vi "System4.vi"() -> ()   [LabVIEW 2013]
uses:
  <vilib>/imath/engines/lvmath/Plug In/_Char/NIMS_CH_character datatype.ctl
  <vilib>/imath/engines/lvmath/Functions/Error Handling/error.ctl
  <vilib>/Analysis/2dsp.llb/Complex FFT.vi
  <vilib>/Analysis/3filter.llb/Equi-Ripple HighPass (DBL).vi
  <instrlib>/niUSRP/niUSRP Fetch Rx Data (CDB).vi
  <vilib>/imath/engines/lvmath2/RunTimeEngine/ErrorHandling/NIMS_Finalize Error.vi
  <vilib>/imath/engines/lvmath2/RunTimeEngine/Managers/WorkSpace/UID Generator.vi
  <vilib>/imath/engines/lvmath2/RunTimeEngine/BuiltInFunctions/length/NIMS_length(GV).vi
  <instcachedir>/0/NIMS_length(GV)_08A3D13377FD4E4B96F5795FBF3698FA.lvgen/NIMS_length(GV)_08A3D13377FD4E4B96F5795FBF3698FA_001.vi
  <vilib>/imath/engines/lvmath2/RunTimeEngine/RangeToken/NIMS_Range_R2 - Integer.vi
  <instcachedir>/0/NIMS_Range_R2 - Integer_C51C130E5EA5464EA148B28CDAB9615A.lvgen/NIMS_Range_R2 - Integer_C51C130E5EA5464EA148B28CDAB9615A_000.vi
  <vilib>/imath/engines/lvmath2/RunTimeEngine/Managers/SymbolTable/Clear UID.vi
  <vilib>/imath/engines/lvmath2/RunTimeEngine/NodeEndStatement/NIMS_NodeEndStatement_Output.vi
  <instcachedir>/0/NIMS_NodeEndStatement_Output_53EC0D466D134D7ABD903AC30B43404B.lvgen/NIMS_NodeEndStatement_Output_53EC0D466D134D7ABD903AC30B43404B_014.vi
  <instcachedir>/0/NIMS_NodeEndStatement_Output_53EC0D466D134D7ABD903AC30B43404B.lvgen/NIMS_NodeEndStatement_Output_53EC0D466D134D7ABD903AC30B43404B_011.vi
  <vilib>/imath/engines/lvmath2/RunTimeEngine/IndexRead/NIMS V(S).vi
  <instcachedir>/0/NIMS V(S)_0488751826AF41519A22953C041130DC.lvgen/NIMS V(S)_0488751826AF41519A22953C041130DC_005.vi
  <vilib>/imathl/engines/lvmath/Functions/Error Handling/Create Error.vi
  <vilib>/imath/engines/lvmath2/RunTimeEngine/BuiltInFunctions/figure/NIMS_figure(I32).vi
  <vilib>/imath/engines/lvmath/Plug In/_Char/NIMS_CH_Character RV to String.vi
  <vilib>/imath/engines/lvmath2/RunTimeEngine/BuiltInFunctions/plot/NIMS_plot(G, Str).vi
  <instcachedir>/0/NIMS_plot(G, Str)_30D49D8623E0484DBD39D394DDFCBE95.lvgen/NIMS_plot(G, Str)_30D49D8623E0484DBD39D394DDFCBE95_000.vi
  <vilib>/imath/engines/lvmath2/RunTimeEngine/NonStaticBuiltInFunctions/Manual/NIMS_NS_load.vi
  <vilib>/imath/engines/lvmath2/RunTimeEngine/RunTimeType/NIMS_RunTimeType_From StrictType (excl LVString).vi
  <instcachedir>/0/NIMS_RunTimeType_From StrictType (excl LVString)_4DEE718D6EB74582AA20236969C084FC.lvgen/NIMS_RunTimeType_From StrictType (excl LVString)_4DEE718D6EB74582AA20236969C084FC_000.vi
  <vilib>/imath/engines/lvmath2/RunTimeEngine/Managers/SymbolTable/Write Variable.vi
  <vilib>/imath/engines/lvmath2/RunTimeEngine/RowToken/NIMS_RowToken-nonstatic.vi
  <vilib>/imath/engines/lvmath2/RunTimeEngine/MatrixToken/NIMS_MatrixToken-nonstatic.vi
  <vilib>/imath/engines/lvmath2/RunTimeEngine/RunTimeSymbolToken/NIMS_RunTimeSymbolToken_ReadVariable-1out.vi
  <vilib>/imath/engines/lvmath/Functions/Error Handling/MergeErrorsWrapper.vi
  <vilib>/imath/engines/lvmath2/RunTimeEngine/LocalVariableDefStatement/MC_LocalVariableDefStatement_Display.vi
  <vilib>/imath/engines/lvmath2/RunTimeEngine/RunTimeSymbolToken/NIMS_RunTimeSymbolToken_ResolveSymbol.vi
  <instcachedir>/0/NIMS_RunTimeSymbolToken_ResolveSymbol_F94DACEDB8D84373A3303A9E667D843C.lvgen/NIMS_RunTimeSymbolToken_ResolveSymbol_F94DACEDB8D84373A3303A9E667D843C_003.vi
  <vilib>/imath/engines/lvmath2/RunTimeEngine/CommandStatement/NIMS_CommandStatement_MaskErr.vi
  <vilib>/imath/engines/lvmath2/RunTimeEngine/Managers/SymbolTable/Read Variable.vi
  <vilib>/imath/engines/lvmath2/RunTimeEngine/RunTimeType/NIMS_RunTimeType_Get Case Value.vi
  <vilib>/imath/engines/lvmath2/RunTimeEngine/NodeEndStatement/MC_NodeEndStatement_Dispose.vi
  <instcachedir>/0/NIMS_NodeEndStatement_Output_53EC0D466D134D7ABD903AC30B43404B.lvgen/NIMS_NodeEndStatement_Output_53EC0D466D134D7ABD903AC30B43404B_004.vi
  <vilib>/imath/engines/lvmath2/RunTimeEngine/RunTimeType/NIMS_RunTimeType_To Numeric.vi
  <instcachedir>/0/NIMS_RunTimeType_To Numeric_4795FB10E831402FABFA341B47E20681.lvgen/NIMS_RunTimeType_To Numeric_4795FB10E831402FABFA341B47E20681_000.vi
  <vilib>/imath/engines/lvmath2/RunTimeEngine/NodeEndStatement/NIMS_NodeEndStatement_Get Vector.vi
  <instcachedir>/0/NIMS_NodeEndStatement_Get Vector_BE4364D373AE46158CA0B14DEB6F98C8.lvgen/NIMS_NodeEndStatement_Get Vector_BE4364D373AE46158CA0B14DEB6F98C8_003.vi
  <vilib>/imath/engines/lvmath/Plug In/_Char/RunTimeType/NIMS_CH_RunTimeType_To Character 2D.vi
  <instcachedir>/0/NIMS_NodeEndStatement_Get Vector_BE4364D373AE46158CA0B14DEB6F98C8.lvgen/NIMS_NodeEndStatement_Get Vector_BE4364D373AE46158CA0B14DEB6F98C8_000.vi
  <vilib>/imath/engines/lvmath/Plug In/_Char/NIMS_CH_Character 1D to U8 1D.vi
  <instcachedir>/0/NIMS_NodeEndStatement_Output_53EC0D466D134D7ABD903AC30B43404B.lvgen/NIMS_NodeEndStatement_Output_53EC0D466D134D7ABD903AC30B43404B_000.vi
  <instcachedir>/0/NIMS_NodeEndStatement_Output_53EC0D466D134D7ABD903AC30B43404B.lvgen/NIMS_NodeEndStatement_Output_53EC0D466D134D7ABD903AC30B43404B_001.vi
  <instcachedir>/0/NIMS_length(GV)_08A3D13377FD4E4B96F5795FBF3698FA.lvgen/NIMS_length(GV)_08A3D13377FD4E4B96F5795FBF3698FA_002.vi
  <vilib>/imath/engines/lvmath2/RunTimeEngine/IndexRead/NIMS V(R2).vi
  <instcachedir>/0/NIMS V(R2)_C76619605A0E4E9F8B2FA9389712AC47.lvgen/NIMS V(R2)_C76619605A0E4E9F8B2FA9389712AC47_001.vi
  <vilib>/imath/engines/lvmath2/RunTimeEngine/BuiltInFunctions/angle/NIMS_angle.vi
  <instcachedir>/0/NIMS_angle_6DDAE2BD99E0421EB990B6436E94D88F.lvgen/NIMS_angle_6DDAE2BD99E0421EB990B6436E94D88F_005.vi
  <vilib>/imath/engines/lvmath2/RunTimeEngine/RangeToken/NIMS_Range.vi
  <instcachedir>/0/NIMS_Range_7481B155BEE341ECA0F59DDB444E2C09.lvgen/NIMS_Range_7481B155BEE341ECA0F59DDB444E2C09_001.vi
  <vilib>/imath/engines/lvmath2/RunTimeEngine/IndexRead/NIMS V(V).vi
  <instcachedir>/0/NIMS V(V)_298D9CB7BFEB42B8BC8D9C3C28AE8C70.lvgen/NIMS V(V)_298D9CB7BFEB42B8BC8D9C3C28AE8C70_000.vi
  <vilib>/imath/engines/lvmath2/RunTimeEngine/BuiltInFunctions/mean/NIMS_CS=mean(CV,I32).vi
  <instcachedir>/0/NIMS_angle_6DDAE2BD99E0421EB990B6436E94D88F.lvgen/NIMS_angle_6DDAE2BD99E0421EB990B6436E94D88F_003.vi
  <vilib>/imath/engines/lvmath2/RunTimeEngine/ErrorHandling/NIMS_Create Error From Enums.vi
  <vilib>/imath/engines/lvmath2/RunTimeEngine/BuiltInFunctions/mean/NIMS_RS=mean(RV,I32).vi
  <vilib>/imath/engines/lvmath2/RunTimeEngine/BuiltInFunctions/abs/NIMS_abs(signed).vi
  <instcachedir>/0/NIMS_abs(signed)_C4FCB8E6058B49B797C7C8D53CA5F6EC.lvgen/NIMS_abs(signed)_C4FCB8E6058B49B797C7C8D53CA5F6EC_000.vi
  <vilib>/imath/engines/lvmath2/RunTimeEngine/BuiltInFunctions/linramp/NIMS_linramp.vi
  <vilib>/imath/engines/lvmath2/RunTimeEngine/ArithmeticOperatorToken/NIMS_ArithmeticOperator_plus.vi
  <instcachedir>/0/NIMS_ArithmeticOperator_plus_8A46DAFC24D445C9B2C97B626139369E.lvgen/NIMS_ArithmeticOperator_plus_8A46DAFC24D445C9B2C97B626139369E_005.vi
  <vilib>/imath/engines/lvmath2/RunTimeEngine/BuiltInFunctions/numelements/NIMS_numelements.vi
  <instcachedir>/0/NIMS_numelements_A776DA77F73142F68C2F209B523114C5.lvgen/NIMS_numelements_A776DA77F73142F68C2F209B523114C5_003.vi
  <vilib>/imath/engines/lvmath2/RunTimeEngine/BuiltInFunctions/zeros/NIMS_V=zeros(I32,I32).vi
  <vilib>/imath/engines/lvmath2/RunTimeEngine/CommandStatement/MC_CommandStatement_break.vi
  LabVIEW Data/MathScriptVIs/MCStatic_31879994332_13cee6d0e2951097849577d15734aa47.vi
  <instcachedir>/0/MCStatic_31879994332_13cee6d0e2951097849577d15734aa47_8B05E9F3DA25454388965366AFABC993.lvgen/MCStatic_31879994332_13cee6d0e2951097849577d15734aa47_8B05E9F3DA25454388965366AFABC993_000.vi
  <vilib>/imath/engines/lvmath2/RunTimeEngine/IndexReplace/NIMS V(S)=S.vi
  <instcachedir>/0/NIMS V(S)=S_66A18068148B4981A312229A93EA5C06.lvgen/NIMS V(S)=S_66A18068148B4981A312229A93EA5C06_001.vi
  <instcachedir>/0/NIMS V(S)=S_66A18068148B4981A312229A93EA5C06.lvgen/NIMS V(S)=S_66A18068148B4981A312229A93EA5C06_000.vi
  <instcachedir>/0/NIMS_plot(G, Str)_30D49D8623E0484DBD39D394DDFCBE95.lvgen/NIMS_plot(G, Str)_30D49D8623E0484DBD39D394DDFCBE95_001.vi
  <vilib>/imath/engines/lvmath2/RunTimeEngine/BuiltInFunctions/title/NIMS_title.vi
  <vilib>/imath/engines/lvmath2/RunTimeEngine/BuiltInFunctions/round/NIMS_round(DBL-S).vi
  <vilib>/imath/engines/lvmath2/RunTimeEngine/BuiltInFunctions/grid/NIMS_grid(Enums).vi
  <instcachedir>/0/NIMS V(S)_0488751826AF41519A22953C041130DC.lvgen/NIMS V(S)_0488751826AF41519A22953C041130DC_000.vi
  <instcachedir>/0/NIMS_abs(signed)_C4FCB8E6058B49B797C7C8D53CA5F6EC.lvgen/NIMS_abs(signed)_C4FCB8E6058B49B797C7C8D53CA5F6EC_001.vi
  <vilib>/imath/engines/lvmath2/RunTimeEngine/BuiltInFunctions/max/1 input/NIMS_max(RV).vi
  <instcachedir>/0/NIMS_max(RV)_237633DB1D604D5BA7001287DF3C7957.lvgen/NIMS_max(RV)_237633DB1D604D5BA7001287DF3C7957_000.vi
  <instcachedir>/0/NIMS_Range_7481B155BEE341ECA0F59DDB444E2C09.lvgen/NIMS_Range_7481B155BEE341ECA0F59DDB444E2C09_000.vi
  <vilib>/imath/engines/lvmath2/RunTimeSupport/NIMS_Error if Not Equal.vi
  <instcachedir>/0/NIMS_Error if Not Equal_902F5D2649E64F5087A1EF57C55C58AB.lvgen/NIMS_Error if Not Equal_902F5D2649E64F5087A1EF57C55C58AB_001.vi
  <vilib>/imath/engines/lvmath2/RunTimeEngine/BuiltInFunctions/repeatmx/NIMS_repeatmx(GM, I32, I32).vi
  <instcachedir>/0/NIMS_repeatmx(GM, I32, I32)_71D32CAC8D434697AB9DA7B55FCB46E4.lvgen/NIMS_repeatmx(GM, I32, I32)_71D32CAC8D434697AB9DA7B55FCB46E4_003.vi
  <vilib>/imath/engines/lvmath2/RunTimeEngine/ArithmeticOperatorToken/NIMS_ArithmeticOperator_minus.vi
  <instcachedir>/0/NIMS_ArithmeticOperator_minus_5462A7974F41415E96B34B7C9D041F4F.lvgen/NIMS_ArithmeticOperator_minus_5462A7974F41415E96B34B7C9D041F4F_008.vi
  <instcachedir>/0/NIMS_abs(signed)_C4FCB8E6058B49B797C7C8D53CA5F6EC.lvgen/NIMS_abs(signed)_C4FCB8E6058B49B797C7C8D53CA5F6EC_003.vi
  <vilib>/imath/engines/lvmath2/RunTimeEngine/BuiltInFunctions/min/1 input/NIMS_min(RM).vi
  <instcachedir>/0/NIMS_min(RM)_0DDFAEBC1781439CA067A573026FA64C.lvgen/NIMS_min(RM)_0DDFAEBC1781439CA067A573026FA64C_000.vi
  <vilib>/imath/engines/lvmath2/RunTimeEngine/IndexRead/NIMS M($,V).vi
  <instcachedir>/0/NIMS M($,V)_706F2CE2C8E141269FD4C8A402E169C5.lvgen/NIMS M($,V)_706F2CE2C8E141269FD4C8A402E169C5_004.vi
  <vilib>/imath/engines/lvmath2/RunTimeEngine/IndexReplace/NIMS M($,V)=M.vi
  <instcachedir>/0/NIMS M($,V)=M_DD8F56E7222B4C7AB43CEE6CDE526A04.lvgen/NIMS M($,V)=M_DD8F56E7222B4C7AB43CEE6CDE526A04_003.vi
  <vilib>/imath/engines/lvmath2/RunTimeEngine/IndexRead/NIMS M($).vi
  <instcachedir>/0/NIMS M($)_82D1177398184AFB96A6AFB63C3C3F57.lvgen/NIMS M($)_82D1177398184AFB96A6AFB63C3C3F57_005.vi
  <vilib>/imath/engines/lvmath2/RunTimeEngine/BuiltInFunctions/hold/NIMS_hold(Enums).vi
  <vilib>/imath/engines/lvmath2/RunTimeEngine/BuiltInFunctions/imag/NIMS_imag(Complex).vi
  <instcachedir>/0/NIMS_imag(Complex)_3180D40D00C843A49C2B33397F857BF3.lvgen/NIMS_imag(Complex)_3180D40D00C843A49C2B33397F857BF3_002.vi
  <instcachedir>/0/MCStatic_31879994332_13cee6d0e2951097849577d15734aa47_8B05E9F3DA25454388965366AFABC993.lvgen/MCStatic_31879994332_13cee6d0e2951097849577d15734aa47_8B05E9F3DA25454388965366AFABC993_002.vi
  <vilib>/imath/engines/lvmath2/RunTimeEngine/BuiltInFunctions/crosscorr/NIMS_crosscorr(GV,GV,Str).vi
  <instcachedir>/0/NIMS_crosscorr(GV,GV,Str)_7F516622EB1B4986A7D0F3F178AC2F2E.lvgen/NIMS_crosscorr(GV,GV,Str)_7F516622EB1B4986A7D0F3F178AC2F2E_000.vi
  <instcachedir>/0/NIMS_abs(signed)_C4FCB8E6058B49B797C7C8D53CA5F6EC.lvgen/NIMS_abs(signed)_C4FCB8E6058B49B797C7C8D53CA5F6EC_006.vi
  LabVIEW Data/MathScriptVIs/MCStatic_31879994332_51ed6d19a1ca34c572878de5410fc211.vi
  <instcachedir>/0/MCStatic_31879994332_51ed6d19a1ca34c572878de5410fc211_95B5E1E0CE2B47CE84A8C3844D693930.lvgen/MCStatic_31879994332_51ed6d19a1ca34c572878de5410fc211_95B5E1E0CE2B47CE84A8C3844D693930_000.vi
  <instcachedir>/0/NIMS V(R2)_C76619605A0E4E9F8B2FA9389712AC47.lvgen/NIMS V(R2)_C76619605A0E4E9F8B2FA9389712AC47_002.vi
  <vilib>/imath/engines/lvmath2/RunTimeEngine/ArithmeticOperatorToken/NIMS_ArithmeticOperator_rightdiv(C,C).vi
  <instcachedir>/0/NIMS_ArithmeticOperator_rightdiv(C,C)_088115A0C99E4A54BFBAA9DF92471D5B.lvgen/NIMS_ArithmeticOperator_rightdiv(C,C)_088115A0C99E4A54BFBAA9DF92471D5B_000.vi
  <instcachedir>/0/NIMS_ArithmeticOperator_minus_5462A7974F41415E96B34B7C9D041F4F.lvgen/NIMS_ArithmeticOperator_minus_5462A7974F41415E96B34B7C9D041F4F_016.vi
  <instcachedir>/0/NIMS_abs(signed)_C4FCB8E6058B49B797C7C8D53CA5F6EC.lvgen/NIMS_abs(signed)_C4FCB8E6058B49B797C7C8D53CA5F6EC_007.vi
  <vilib>/imath/engines/lvmath2/RunTimeEngine/BuiltInFunctions/sum/NIMS_sum(GV).vi
  <instcachedir>/0/NIMS_sum(GV)_67F5EC36BC034E54A6BEC5B0673C00E5.lvgen/NIMS_sum(GV)_67F5EC36BC034E54A6BEC5B0673C00E5_000.vi
  MATLAB_func/frequency_synchronisation_sample.m
  MATLAB_func/quadrature_error_correction.m
  <vilib>/imath/engines/lvmath2/RunTimeEngine/Managers/SymbolTable/NIMS_WorkSpace.lvlib
  <vilib>/Analysis/NI_AALPro.lvlib
  <vilib>/Analysis/NI_AALBase.lvlib
  <instcachedir>/0/MCStatic_31879994332_13cee6d0e2951097849577d15734aa47_8B05E9F3DA25454388965366AFABC993.lvgen/MCStatic_31879994332_13cee6d0e2951097849577d15734aa47_8B05E9F3DA25454388965366AFABC993_003.vi
panel:
  out "coerced carrier frequency":dbl=100000.0 format="%#_6p"
  out "Waveform Graph 6":dbl[](graph)
  out "bit_error_rate":dbl
  out "error":dbl
  out "size(s)":i32
  out "length_signal_out":i32
  in  "file (use dialog) 2":path=path "C:/Users/Lab/Downloads/FPGA.3JPG"
  in  "file (use dialog)":path=path "C:/Users/Lab/Downloads/FPGA.JPG"
  out "time":dbl
  out "a":cdb[](array[numeric])
  in  "message number of samples (50000)":i64=50000
  in  "stop 2":bool
  in  "Wakeup #samples (1000)":i64=1000
  out "RX coerced gain":dbl format="%#_6f"
  out "RX coerced IQ rate":dbl=100000.0 format="%#_6p"
  in  "RX gain":dbl format="%#_6f"
  in  "RX IQ rate":dbl=1000000.0 format="%#_6p"
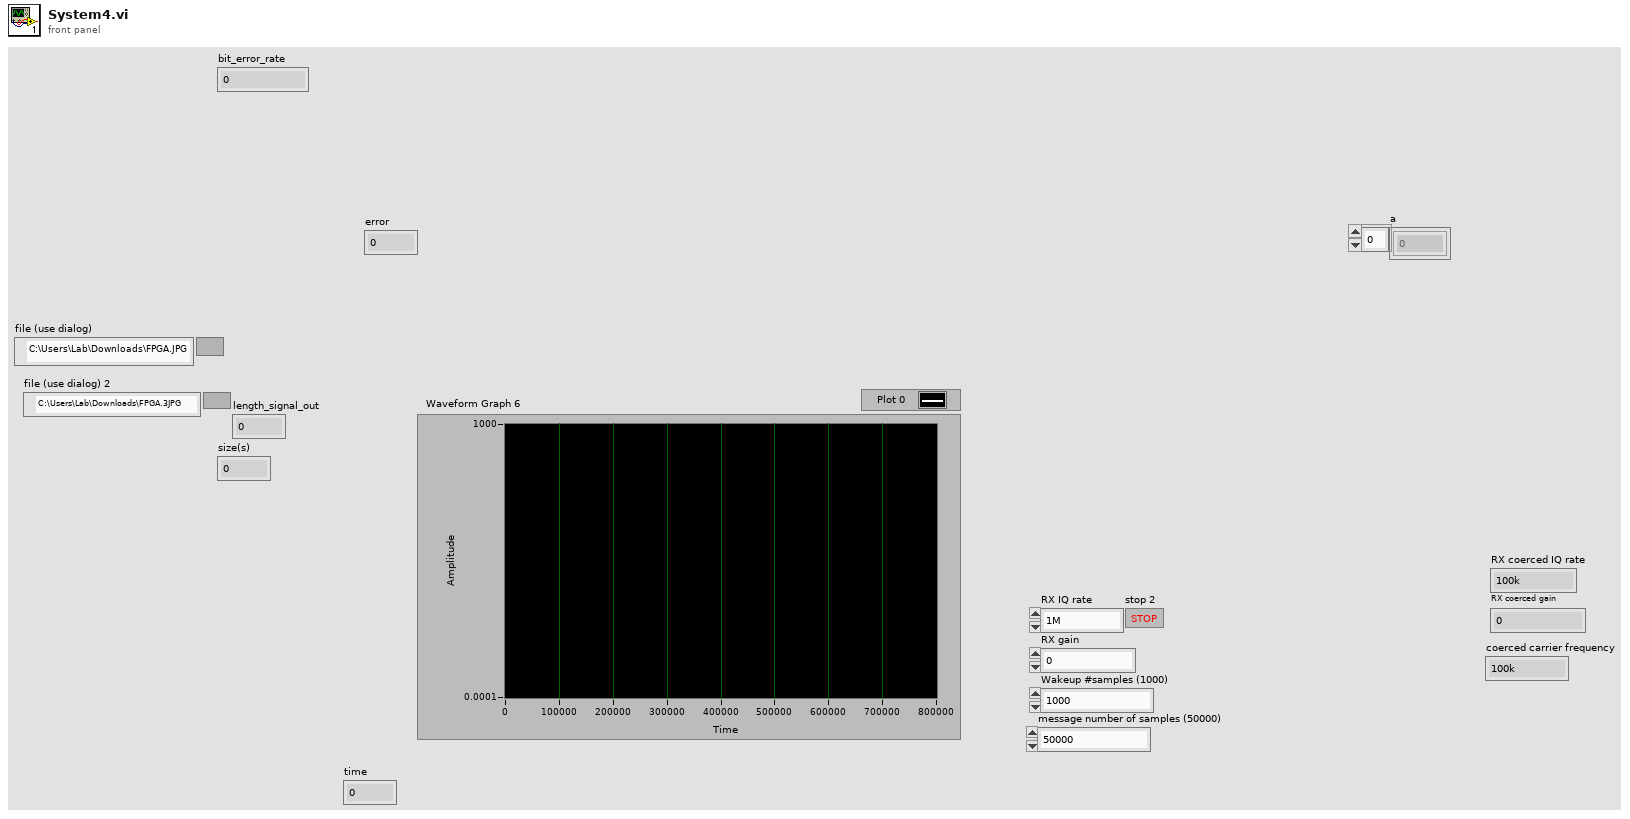
[diagram p1: front panel]
types:
  T1 = typedef "NIMS_CH_character datatype.ctl" = cluster{"Numeric":u8}
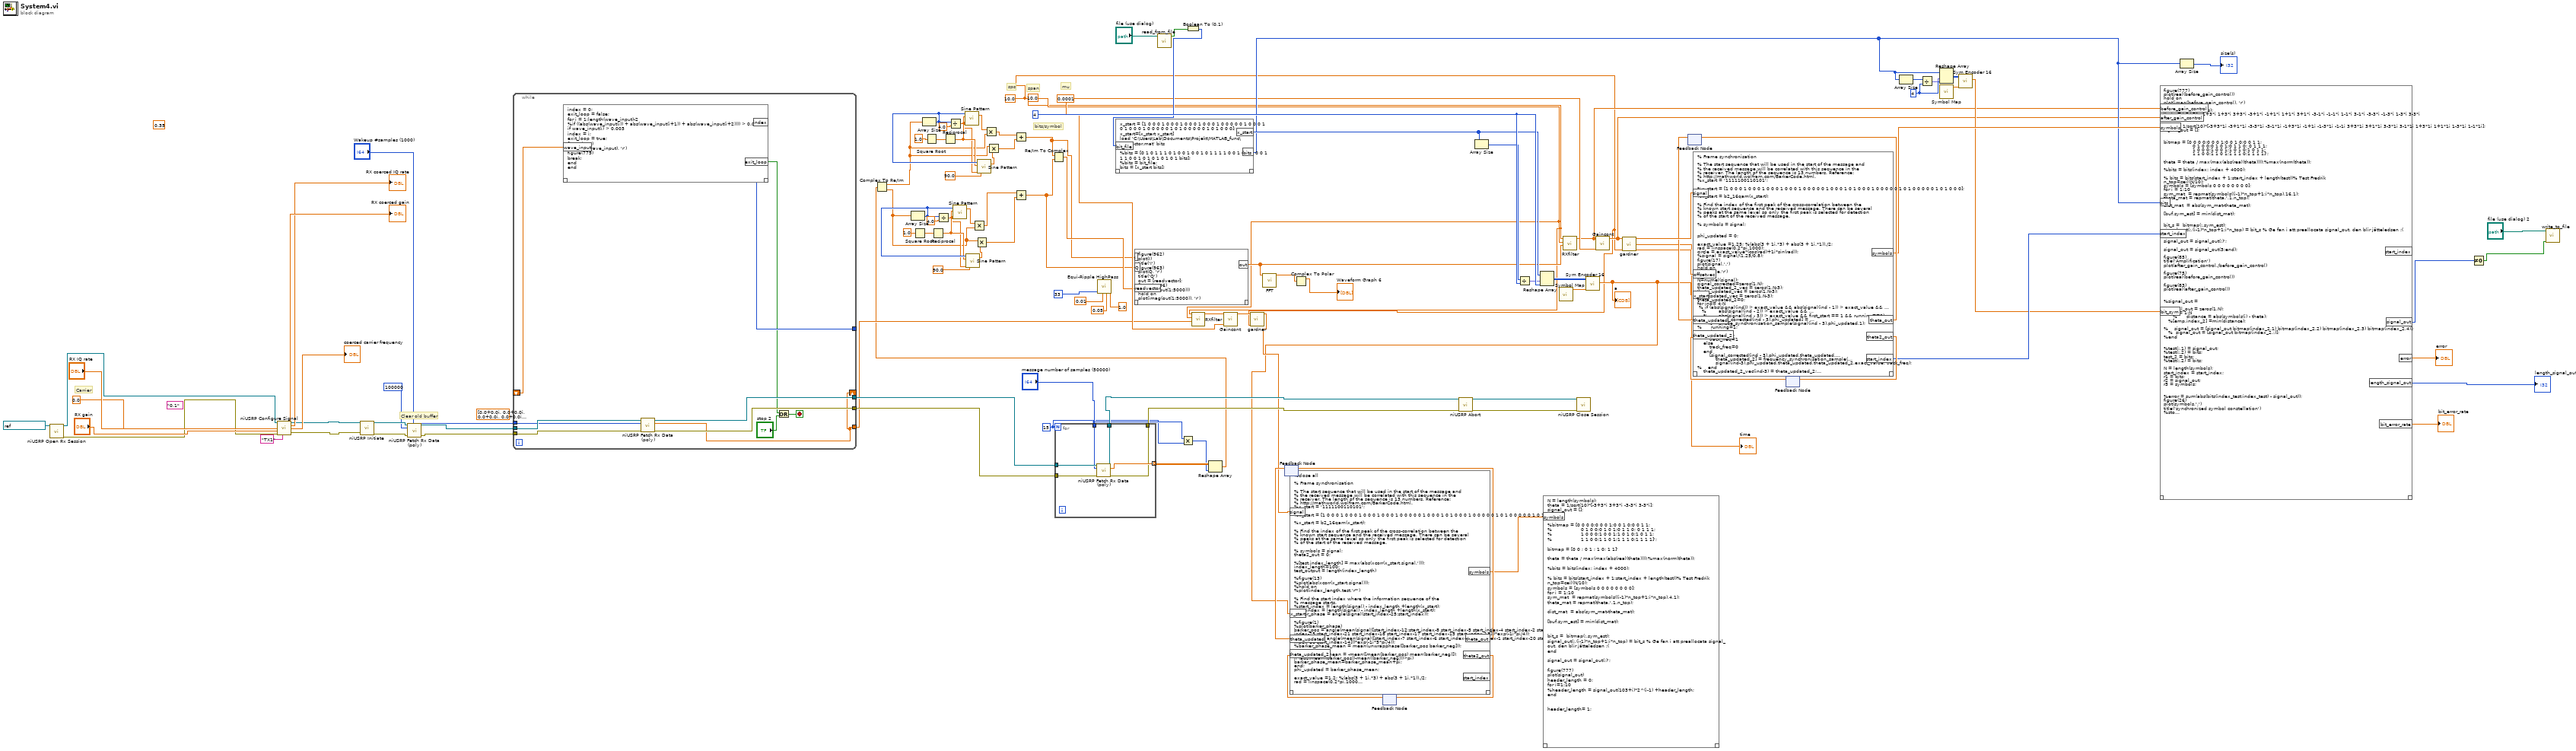
[diagram p0: block diagram]
diagram:
  (unwired) "0,1" ("Configuration:Enabled Channels")
  (unwired) 0.35 ("a")
  (unwired) cdb[] [0.0+0.0i, 0.0+0.0i, 0.0+0.0i, 0.0+0.0i, 0.0+0.0i, 0.0+0.0i, 0.0+0.0i, 0.0+0.0i, 0.0+0.0i, 0.0+0.0i, 0.0+0.0i, 0.0+0.0i, 0.0+0.0i, 0.0+0.0i, 0.0+0.0i, 0.0+0.0i, 0.0+0.0i] ("data")
  w67 = 4 ("dimension size")
  w79 = 15
  w45 = 10.0 ("span")
  w104 = 4 ("dimension size")
  w59 = 0.0001 ("mu")
  w46 = 10.0 ("span")
  # "Clear old buffer"
  # "sps"
  # "bits/symbol"
  # "span"
  # "mu"
  # "Carrier"
  n1 = call <instrlib>:"niUSRP Open Rx Session.vi"("device names"=refnum<k15> "192.168.10.9") -> ("session handle out"=w30:refnum<k15>, "error out"=w31:errorcluster)  [unwired: 13 in]
  n2 = call <instrlib>:"niUSRP Configure Signal.vi"("session handle"=w30, "IQ rate"="RX IQ rate", "carrier frequency"=0.0, "gain"="RX gain", "error in (no error)"=w31, "active antenna"="TX1") -> ("session handle out"=w33:refnum<k15>, "coerced IQ rate"=→"RX coerced IQ rate":dbl, "coerced carrier frequency"=→"coerced carrier frequency":dbl, "coerced gain"=→"RX coerced gain":dbl, "error out"=w32:errorcluster)  [unwired: 5 in]
  n3 = call <instrlib>:"niUSRP Initiate.vi"("session handle"=w33, "error in (no error)"=w32) -> ("session handle out"=w88:refnum<k15>, "error out"=w89:errorcluster)  [unwired: 12 in]
  n4 = call-poly <instrlib>:"niUSRP Fetch Rx Data (poly).vi"("session handle"=w88, "number of samples"=i64 100000, "error in (no error)"=w89) -> ("session handle out"=w91:refnum<k15>, "error out"=w90:errorcluster)  [unwired: 9 in, 2 out]
  n5 = while {
    tunnel: w91 -> [w121]
    tunnel: w90 -> [w120]
    tunnel: [w119] -> w86
    tunnel: [w118] -> w85
    tunnel: "Wakeup #samples (1000)" -> [w117]
    tunnel: [w116] -> _
    shift-right: [w112] -> _
    shift-left: _ -> [w111]
    tunnel: [w112] -> w23
    stop <- w114 stop-if-true
    n6 = mathscript code="index = 0;\nexit_loop = false;\nfor i = 1:length(wave_input)-2\n%if ((abs(wave_input(i)) + abs(wave_input(i+1)) + abs(wave_input(i+2)))) > 0.002\nif wave_input(i) > 0.003\nindex = i;\nexit_loop = true;\nfigure(123)\nplot(real(wave_input), 'r')\nfigure(779)\nbreak;\nend\nend"("wave_input"=w111) -> ("index"=w116:i32, "exit_loop"=w113:bool)  [unwired: 1 in, 1 out]
    n7 = call-poly <instrlib>:"niUSRP Fetch Rx Data (poly).vi"("session handle"=w121, "number of samples"=w117, "error in (no error)"=w120) -> ("session handle out"=w119:refnum<k15>, "data"=w112:cdb[], "error out"=w118:errorcluster)  [unwired: 9 in, 1 out]
    n8 = Or(x=w113, y="stop 2") -> (x .or. y?=w114:bool)
  }
  n9 = Square Root(x=1.0) -> (sqrt(x)=w14:dbl)
  n10 = Square Root(x=1.0) -> (sqrt(x)=w27:dbl)
  n11 = Reciprocal(x=w14) -> (1/x=w9:dbl)
  n12 = Reciprocal(x=w27) -> (1/x=w20:dbl)
  n13 = for {
    N: w79 -> [_]
    tunnel: w86 -> [w323]
    tunnel: w85 -> [w322]
    tunnel: [w321] -> w84 mode=indexing
    tunnel: "message number of samples (50000)" -> [w320]
    tunnel: [w319] -> w83
    tunnel: [w318] -> w82
    n14 = call-poly <instrlib>:"niUSRP Fetch Rx Data (poly).vi"("session handle"=w323, "number of samples"=w320, "error in (no error)"=w322) -> ("session handle out"=w319:refnum<k15>, "data"=w321:cdb[], "error out"=w318:errorcluster)  [unwired: 9 in, 1 out]
  }
  n15 = call-poly <vilib>:"Equi-Ripple HighPass.vi"("# of taps"=33, "stop freq"=0.01, "high freq"=0.05, "sampling freq: fs"=1.0) -> ()  [unwired: 2 in, 2 out]
  n16 = call "read_from_file.vi"("file (use dialog)"="file (use dialog)") -> ("data"=w76:bool[])  [unwired: 10 in]
  n17 = Multiply(x="message number of samples (50000)", y=w79) -> (x*y=w81:i64)
  n18 = Boolean To (0,1)(Boolean=w76) -> (0, 1=w75:i16[])
  n19 = mathscript code="x_start = [1 0 0 0 1 0 0 0 1 0 0 0 1 0 0 0 1 0 0 0 0 0 1 0 0 0 1 0 1 0 0 0 1 0 0 0 0 0 1 0 1 0 0 0 0 0 1 0 1 0 0 0];\nx_start=[x_start x_start]\nload 'C:\\Users\\Lab\\Documents\\Projekt\\MATLAB_func\\testvector.mat' bits\n\n%bits = [0 1 0 1 1 1 0 1 0 0 1 0 0 1 0 1 1 1 1 0 0 1 0 1 0 0 0 1 1 1 0 0 1 0 1 0 1 0 1 0 1 bits];\n%bits = bit_file;\nbits = [x_start bits];"("bit_file"=w75) -> ("x_start"=w100:i32[], "bits"=w64:i32[])  [unwired: 1 in, 1 out]
  n20 = call "RXfilter.vi"("Array"=w23, "span"=w46, "sps"=w45) -> ("out"=w60:cdb[])  [unwired: 8 in]
  n21 = Reshape Array(w84, w81) -> (w22:cdb[])
  n22 = Complex To Re/Im(x + iy=w22) -> (x=w18:dbl[], y=w7:dbl[])
  n23 = Array Size(array=w7) -> (size(s)=w10:i32)
  n24 = Array Size(array=w18) -> (size(s)=w21:i32)
  n25 = Divide(x=w10, y=4.0) -> (x/y=w8:dbl)
  n26 = Divide(x=w21, y=4.0) -> (x/y=w19:dbl)
  n27 = call <vilib>:"Sine Pattern.vi"("cycles"=w8, "amplitude"=w9, "samples"=w10) -> ("Sinusoidal Pattern"=w12:dbl[])  [unwired: 1 in, 1 out]
  n28 = call <vilib>:"Sine Pattern.vi"("cycles"=w19, "amplitude"=w20, "samples"=w21) -> ("Sinusoidal Pattern"=w25:dbl[])  [unwired: 1 in, 1 out]
  n29 = call <vilib>:"Sine Pattern.vi"("cycles"=w8, "phase(degrees)"=90.0, "amplitude"=w9, "samples"=w10) -> ("Sinusoidal Pattern"=w11:dbl[])  [unwired: 1 out]
  n30 = Multiply(x=w12, y=w7) -> (x*y=w3:dbl[])
  n31 = Multiply(x=w7, y=w11) -> (x*y=w4:dbl[])
  n32 = call <vilib>:"Sine Pattern.vi"("cycles"=w19, "phase(degrees)"=90.0, "amplitude"=w20, "samples"=w21) -> ("Sinusoidal Pattern"=w24:dbl[])  [unwired: 1 out]
  n33 = Multiply(x=w25, y=w18) -> (x*y=w6:dbl[])
  n34 = Multiply(x=w18, y=w24) -> (x*y=w5:dbl[])
  n35 = Add(x=w6, y=w5) -> (x+y=w2:dbl[])
  n36 = Add(x=w3, y=w4) -> (x+y=w1:dbl[])
  n37 = Re/Im To Complex(1:w1, 2:w2) -> (0:w17:cdb[])
  n38 = mathscript code="figure(962)\nplot(I)\ntitle('I')\nfigure(963)\nplot(Q, 'r')\ntitle('Q')\nout = [readvector];\nfigure(9996)\nplot(real(out(1:5000)))\nhold on\nplot(imag(out(1:5000)), 'r')"("readvector"=w17, "I"=w2, "Q"=w1) -> ("out"=w50:cdb[])  [unwired: 1 in, 1 out]
  n39 = call "Gaincont.vi"("mu"=w59, "Array"=w60) -> ("out"=w61:cdb[])  [unwired: 9 in]
  n40 = call "gardner.vi"("in"=w61, "sps"=w45) -> ("sym"=w54:cdb[])  [unwired: 11 in, 2 out]
  n41 = call-poly <vilib>:"FFT.vi"("X"=w50) -> ("FFT {X}"=w39:cdb[])  [unwired: 9 in, 1 out]
  n42 = feedback #1() -> (w55:dbl)  [unwired: 1 in]
  n43 = Complex To Polar(r * e^(i*theta)=w39) -> (r=→"Waveform Graph 6":dbl[])  [unwired: 1 out]
  n44 = feedback #2() -> (w57:dbl)  [unwired: 1 in]
  n45 = call <instrlib>:"niUSRP Abort.vi"("session handle"=w83, "error in (no error)"=w82) -> ("session handle out"=w109:refnum<k15>, "error out"=w108:errorcluster)  [unwired: 12 in]
  n46 = Array Size(array=w100) -> (size(s)=w101:i32)
  n47 = Divide(x=w101, y=w104) -> (x/y=w103:fxp<+,27,27>)
  n48 = Reshape Array(w100, w103, w104) -> (w102:i32[][])
  n49 = call "Symbol Map.vi"() -> ("symbol_map"=w105:cdb[])  [unwired: 11 in]
  n50 = call "RXfilter.vi"("Array"=w50, "span"=w46, "sps"=w45) -> ("out"=w49:cdb[])  [unwired: 8 in]
  n51 = call <instrlib>:"niUSRP Close Session.vi"("session handle"=w109, "error in (no error)"=w108) -> ()  [unwired: 13 in, 1 out]
  n52 = call "Sym Encoder 16.vi"("symbol_map"=w105, "b"=w102) -> ("a"=w53:cdb[])  [unwired: 9 in]
  "a" <- w53
  n53 = mathscript code="%close all\n\n% Frame synchronisation\n\n% The start sequence that will be used in the start of the message and\n% the received message will be correlated with this sequence in the \n% receiver. The length of the sequence is 13 numbers. Reference: \n% http://mathworld.wolfram.com/BarkerCode.html.\n%x_start = '1111100110101';\n\n%x_start = [1 0 0 0 1 0 0 0 1 0 0 0 1 0 0 0 1 0 0 0 0 0 1 0 0 0 1 0 1 0 0 0 1 0 0 0 0 0 1 0 1 0 0 0 0 0 1 0 1 0 0 0];\n\n%x_start = b2_16qam(x_start);\n\n% Find the index of the first peak of the cross-correlation between the \n% known start sequence and the received message. There can be several \n% peaks at the same level so only the first peak is selected for detection \n% of the start of the received message.\n\n% symbols = signal;\ntheta2_out = 0;\n\n%[test,index_length] = max(abs(xcorr(x_start,signal.')));\nindex_length=100;\ntest_output = length(index_length)\n\n%figure(13)\n%plot(abs(xcorr(x_start,signal)));\n%hold on\n%plot(index_length,test,'r*')\n\n% Find the start index where the information sequence of the \n% message starts.\n%start_index = length(signal) - index_length +length(x_start);\nstart_index = length(signal) - index_length +length(x_start);\nbarker_phase = angle(signal(start_index-25:start_index));\n\n%figure(1)\n%plot(barker_phase)\nbarker_pos = angle(mean(signal([start_index-12:start_index-8 start_index-5 start_index-4 start_index-2 start_index start_index-25:start_index-21 start_index-18 start_index-17 start_index-15 start_index-13]))*exp(-1i*pi/4)); \nbarker_neg = angle(mean(signal([start_index-7 start_index-6 start_index-3 start_index-1 start_index-20 start_index-19 start_index-16 start_index-14]))*exp(-1i*5*pi/4)); \n%barker_phase_mean = mean(unwrapphase([barker_pos barker_neg]));\n\nbarker_phase_mean = -mean([mean(barker_pos) mean(barker_neg)]);\nif (abs(mean((barker_pos))-mean((barker_neg)))>pi)\nbarker_phase_mean=barker_phase_mean+pi;\nend;\nphi_updated = barker_phase_mean;\n\nexact_value =1.2; %(abs(3 + 1i.*3) + abs(3 + 1i.*1))./2;\nrad = linspace(0,2*pi,1000);\ncircle = exact_value*(cos(rad)+1i*sin(rad));\n%signal = signal/(1.25/0.8);\nN=numel(signal);\nsignal_corrected=zeros(1,N);\ntheta_updated_2_vec = zeros(1,N);\ntheta_updated_vec = zeros(1,N);\nphi_updated_vec = zeros(1,N);\n\nfor ind= 4:N\n % if (abs(signal(ind)) > exact_value && abs(signal(ind - 1)) > exact_value && ...\n   %        abs(signal(ind - 2)) > exact_value && ...\n    %       abs(signal(ind - 3)) > exact_value && first_start == 1 && running==0)\n      % [signal_corrected(ind - 3),phi_updated] = ...\n       %    phase_synchronisation_sample(signal(ind - 3),phi_updated,1);\n%      running=1;\n   % else\n        [signal_corrected(ind - 3),phi_updated,theta_updated,...\n            theta_updated_2] = frequency_synchronisation_sample(...\n            signal(ind-3),phi_updated,theta_updated,theta_updated_2,exact_value);\n%    end\n    theta_updated_2_vec(ind-3) = theta_updated_2;\n    theta_updated_vec(ind-3) = theta_updated;\n    phi_updated_vec(ind-3) = phi_updated;\n    if (ind == N)\n        for a = 1:3\n            [signal_corrected(N - 3 + a),phi_updated,theta_updated,theta_updated_2] = ...\n                frequency_synchronisation_sample(signal(N - 3 + a),...\n                phi_updated,theta_updated,theta_updated_2,exact_value);\n        end\n    end\n\nend\nplot(signal_corrected(1:end),'.')\ntitle('denna')\ntest_rotation = angle(signal_corrected(1));\n%barker_pos = angle(signal_corrected([start_index-12:start_index-8 start_index-5 start_index-4 start_index-2 start_index])*exp(-1i*pi/4)); \n%barker_neg = angle(signal_corrected([start_index-7 start_index-6 start_index-3 start_index-1])*exp(-1i*5*pi/4)); \nbarker_pos = angle(mean(signal_corrected([start_index-12:start_index-8 start_index-5 start_index-4 start_index-2 start_index start_index-25:start_index-21 start_index-18 start_index-17 start_index-15 start_index-13]))*exp(-1i*pi/4)); \nbarker_neg = angle(mean(signal_corrected([start_index-7 start_index-6 start_index-3 start_index-1 start_index-20 start_index-19 start_index-16 start_index-14]))*exp(-1i*5*pi/4)); \n%barker_phase_mean = mean(unwrapphase([barker_pos barker_neg]));\n%barker_pos=unwrapphase(barker_pos)\n%barker_neg=unwrapphase(barker_neg)\nbarker_phase_mean = -mean([mean(barker_pos) mean(barker_neg)]);\nif (abs(mean((barker_pos))-mean((barker_neg)))>pi)\nbarker_phase_mean=barker_phase_mean+pi;\nend\ntest_phase = barker_phase_mean;\n\n% barker_phase_mean = mean(unwrapphase(barker_pos));\nphi_updated_2 = barker_phase_mean;\nphi_updated_2 =round(phi_updated_2./(pi/2))*pi/2;\n\n% Test Fredrik and Fredrik\n% symbols = signal_corrected(start_index + 1:start_index + 5000).*exp(1i*phi_updated_2);\nstop = length(signal_corrected(start_index + 1:end));\n\nsymbols = signal_corrected(1:stop).*exp(1i*phi_updated_2);\n\nsymbols = symbols(start_index  - 25:end);\n%symbols = signal_corrected;\nfigure(1337)\nplot(symbols(1:end-1),'.')\ngrid on\nphi_out=phi_updated_vec(N-4);\ntheta_out=theta_updated_vec(N-5);\ntheta2_out=theta_updated_2_vec(N-4);"("x_start"=w53, "signal"=w54, "theta_updated_2"=w57, "theta_updated"=w55) -> ("theta2_out"=w58:dbl, "theta_out"=w56:dbl, "symbols"=w52:cdb[])  [unwired: 1 in, 2 out]
  n54 = feedback-in #1(w56) -> ()
  n55 = feedback-in #2(w58) -> ()
  n56 = mathscript code="N = length(symbols);\ntheta = 1/sqrt(10)*[-3+3*i 3+3*i -3-3*i 3-3*i];\nsignal_out = [];\n\n\n%bitmap = [0 0 0 0;0 0 0 1;0 0 1 0;0 0 1 1;\n%                   0 1 0 0;0 1 0 1;0 1 1 0; 0 1 1 1;\n%                   1 0 0 0;1 0 0 1;1 0 1 0;1 0 1 1;\n%                   1 1 0 0;1 1 0 1;1 1 1 0;1 1 1 1]';\n\nbitmap = [0 0 ; 0 1 ; 1 0; 1 1]'\n\ntheta = theta / max(max(abs(real(theta))));%max(norm(theta));\n\n%bits = bits(index: index + 4000);\n\n% bits = bits(start_index + 1:start_index + length(test))% Test Fredrik\nn_top=ceil(N/10);\nsymbols = [symbols 0 0 0 0 0 0 0 0];\nfor i = 1:10\nsym_mat  = repmat(symbols((i-1)*n_top+1:i*n_top),4,1);\ntheta_mat = repmat(theta.',1,n_top);\n\ndist_mat  = abs(sym_mat-theta_mat);\n\n[buf,sym_est] = min(dist_mat);\n\n\nbit_s =  bitmap(:,sym_est);\nsignal_out(:,(i-1)*n_top+1:i*n_top) = bit_s % Ge fan i att preallocata signal_out, den blir jätteledsen :(\nend\n\nsignal_out = signal_out(:)';\n\nfigure(777)\nplot(signal_out)\nheader_length = 0;\nfor i=1:10\n%header_length = signal_out(103+i)*2^(i-1) +header_length;\nend\n\n\nheader_length= 1;"("symbols"=w52) -> ()  [unwired: 1 in, 1 out]
  n57 = call "Gaincont.vi"("mu"=w59, "Array"=w49) -> ("out"=w48:cdb[])  [unwired: 9 in]
  n58 = call "gardner.vi"("in"=w48, "sps"=w45) -> ("sym"=w99:cdb[], "time"=→"time":dbl, "offsetvec"=w92:dbl[])  [unwired: 11 in]
  n59 = feedback #3() -> (w95:dbl)  [unwired: 1 in]
  n60 = feedback #4() -> (w97:dbl)  [unwired: 1 in]
  n61 = mathscript code="% Frame synchronisation\n\n% The start sequence that will be used in the start of the message and\n% the received message will be correlated with this sequence in the \n% receiver. The length of the sequence is 13 numbers. Reference: \n% http://mathworld.wolfram.com/BarkerCode.html.\n%x_start = '1111100110101';\n\n%x_start = [1 0 0 0 1 0 0 0 1 0 0 0 1 0 0 0 1 0 0 0 0 0 1 0 0 0 1 0 1 0 0 0 1 0 0 0 0 0 1 0 1 0 0 0 0 0 1 0 1 0 0 0];\n\n%x_start = b2_16qam(x_start);\n\n% Find the index of the first peak of the cross-correlation between the \n% known start sequence and the received message. There can be several \n% peaks at the same level so only the first peak is selected for detection \n% of the start of the received message.\n\n% symbols = signal;\n\n\nphi_updated = 0;\n\nexact_value =1.25; %(abs(3 + 1i.*3) + abs(3 + 1i.*1))./2;\nrad = linspace(0,2*pi,1000);\ncircle = exact_value*(cos(rad)+1i*sin(rad));\n%signal = signal/(1.25/0.8);\nfigure(17)\nplot(signal,'.')\nhold on\nplot(circle,'r')\n\nN=numel(signal);\nsignal_corrected=zeros(1,N);\ntheta_updated_2_vec = zeros(1,N-3);\ntheta_updated_vec = zeros(1,N-3);\nphi_updated_vec = zeros(1,N-3);\ntheta_updated_2=0;\nfor ind= 4:N\n % if (abs(signal(ind)) > exact_value && abs(signal(ind - 1)) > exact_value && ...\n   %        abs(signal(ind - 2)) > exact_value && ...\n    %       abs(signal(ind - 3)) > exact_value && first_start == 1 && running==0)\n      % [signal_corrected(ind - 3),phi_updated] = ...\n       %    phase_synchronisation_sample(signal(ind - 3),phi_updated,1);\n%      running=1;\n   % else\n    if ind<10000\n        track_freq=1\n    else\n        track_freq=0\n    end\n        [signal_corrected(ind - 3),phi_updated,theta_updated,...\n            theta_updated_2] = frequency_synchronisation_sample(...\n            signal(ind-3),phi_updated,theta_updated,theta_updated_2,exact_value, track_freq);\n%    end\n    theta_updated_2_vec(ind-3) = theta_updated_2;\n    theta_updated_vec(ind-3) = theta_updated;\n    phi_updated_vec(ind-3) = phi_updated;\n    if (ind == N)\n        for a = 1:3\n            [signal_corrected(N - 3 + a),phi_updated,theta_updated,theta_updated_2] = ...\n                frequency_synchronisation_sample(signal(N - 3 + a),...\n                phi_updated,theta_updated,theta_updated_2,exact_value, track_freq);\n        end\n    end\n   %theta2_out = min(abs(theta_updated_2),1000 )*sign(theta_updated_2)\nend\n%stop=round(length(signal)/4)\nstop=20000;\ntest = abs(xcorr(x_start,signal(1:stop).'));\n%test=[zeros(1, 30) 1]\n\n[test_2,index_length] = max(test);\n\nfigure(553)\nplot(test)\n\ntest_output = length(index_length)\n\n%figure(13)\n%plot(abs(xcorr(x_start,signal)));\n%hold on\n%plot(index_length,test,'r*')\n\n% Find the start index where the information sequence of the \n% message starts.\n%start_index = length(signal) - index_length +length(x_start);%+13;\nfigure(82)\nplot(signal(2000:2010),'.')\nstart_index = stop - index_length +length(x_start);\nreference=[signal_corrected(start_index-1:start_index+2)]\nsignal_corrected=quadrature_error_correction(signal_corrected.', reference.')\n\nfigure(450)\nplot(signal(start_index - 25:start_index),'.')\nfigure(451)\nplot(real(signal(start_index -25:start_index)),'.')\nhold on\nplot(imag(signal(start_index -25:start_index)),'r.')\n\nfigure(81)\nplot(signal_corrected(1000:1004),'.')\nfigure(987)\nplot(signal_corrected(start_index - 25:start_index),'.')\nfigure(28)\nplot(signal_corrected(1:end),'.')\ntest_rotation = angle(signal_corrected(1));\nfigure(452)\nplot(real(signal_corrected(start_index -25:start_index)),'.')\nhold on\nplot(imag(signal_corrected(start_index -25:start_index)),'r.')\n%barker_pos = angle(signal_corrected([start_index-12:start_index-8 start_index-5 start_index-4 start_index-2 start_index])*exp(-1i*pi/4)); \n%barker_neg = angle(signal_corrected([start_index-7 start_index-6 start_index-3 start_index-1])*exp(-1i*5*pi/4)); \nbarker_pos = angle(mean(signal_corrected([start_index-12:start_index-8 start_index-5 start_index-4 start_index-2 start_index start_index-25:start_index-21 start_index-18 start_index-17 start_index-15 start_index-13]))*exp(-1i*pi/4)); \nbarker_neg = angle(mean(signal_corrected([start_index-7 start_index-6 start_index-3 start_index-1 start_index-20 start_index-19 start_index-16 start_index-14]))*exp(-1i*5*pi/4)); \n%barker_phase_mean = mean(unwrapphase([barker_pos barker_neg]));\n%barker_pos=unwrapphase(barker_pos)\n%barker_neg=unwrapphase(barker_neg)\nbarker_phase_mean = -mean([mean(barker_pos) mean(barker_neg)]);\nif (abs(mean((barker_pos))-mean((barker_neg)))>pi)\nbarker_phase_mean=barker_phase_mean+pi;\nend\ntest_phase = barker_phase_mean;\n\n% barker_phase_mean = mean(unwrapphase(barker_pos));\nphi_updated_2 = barker_phase_mean;\nphi_updated_2 =round(phi_updated_2./(pi/2))*pi/2;\n\n% Test Fredrik and Fredrik\n% symbols = signal_corrected(start_index + 1:start_index + 5000).*exp(1i*phi_updated_2);\n%stop = length(signal_corrected(start_index + 1:end));\n\nsymbols = signal_corrected.*exp(1i*phi_updated_2);\n\n\nfigure(455)\ntitle('Barker sequence after synchronisation.')\nplot(real(symbols(start_index -25:start_index)),'.')\nhold on\nplot(imag(symbols(start_index -25:start_index)),'r.')\n\n\n\nsymbols = symbols(start_index  - 25:end);\n%symbols = signal_corrected;\n\nfigure(401)\nplot(real(symbols))\n\nphi_out=phi_updated_vec(N-4);\ntheta_out=theta_updated_vec(N-5);\ntheta2_out=theta_updated_2_vec(N-4);\nfigure(8889)\nplot(theta_updated_vec)\ntitle('Frequency phase correction step size');\nfigure(8888)\nplot(theta_updated_2_vec)\ntitle('Accumulated frequency phase correction');\nfigure(479)\nplot(phi_updated_vec)\ntitle('Phase offset per symbol');\nhold off\nfigure(1337)\nplot(symbols(1:end-1),'.')\ngrid on"("x_start"=w53, "signal"=w99, "theta_updated_2"=w97, "theta_updated"=w95, "offsetvec"=w92) -> ("theta2_out"=w98:dbl, "theta_out"=w96:dbl, "start_index"=w94:i32, "symbols"=w93:cdb[])  [unwired: 1 in, 1 out]
  n62 = feedback-in #3(w96) -> ()
  n63 = feedback-in #4(w98) -> ()
  n64 = Array Size(array=w64) -> (size(s)=w65:i32)
  n65 = Divide(x=w65, y=w67) -> (x/y=w66:fxp<+,27,27>)
  n66 = Reshape Array(w64, w66, w67) -> (w68:i32[][])
  n67 = call "Symbol Map.vi"() -> ("symbol_map"=w69:cdb[])  [unwired: 11 in]
  n68 = call "Sym Encoder 16.vi"("symbol_map"=w69, "b"=w68) -> ("a"=w63:cdb[])  [unwired: 9 in]
  n69 = mathscript code="figure(777)\nplot(real(before_gain_control))\nhold on \nplot(imag(before_gain_control), 'r')\n%symbols\nN = length(symbols);\ntheta = [-3+3*i -1+3*i 1+3*i 3+3*i -3+1*i -1+1*i 1+1*i 3+1*i -3-1*i -1-1*i 1-1*i 3-1*i -3-3*i -1-3*i 1-3*i 3-3*i\n               ];\n\ntheta = 1/sqrt(10)*[-3+3*1i -3+1*1i -3-3*1i -3-1*1i -1+3*1i -1+1i -1-3*1i -1-1i 3+3*1i 3+1*1i 3-3*1i 3-1*1i 1+3*1i 1+1*1i 1-3*1i 1-1*1i];\nsignal_out = [];\n\n\nbitmap = [0 0 0 0;0 0 0 1;0 0 1 0;0 0 1 1;\n                   0 1 0 0;0 1 0 1;0 1 1 0; 0 1 1 1;\n                   1 0 0 0;1 0 0 1;1 0 1 0;1 0 1 1;\n                   1 1 0 0;1 1 0 1;1 1 1 0;1 1 1 1]';\n\ntheta = theta / max(max(abs(real(theta))));%max(norm(theta));\n\n%bits = bits(index: index + 4000);\n\n% bits = bits(start_index + 1:start_index + length(test))% Test Fredrik\nn_top=ceil(N/10);\nsymbols = [symbols 0 0 0 0 0 0 0 0];\nfor i = 1:10\nsym_mat  = repmat(symbols((i-1)*n_top+1:i*n_top),16,1);\ntheta_mat = repmat(theta.',1,n_top);\n\ndist_mat  = abs(sym_mat-theta_mat);\n\n[buf,sym_est] = min(dist_mat);\n\n\nbit_s =  bitmap(:,sym_est);\nsignal_out(:,(i-1)*n_top+1:i*n_top) = bit_s % Ge fan i att preallocata signal_out, den blir jätteledsen :(\nend\n\nsignal_out = signal_out(:)';\n\nsignal_out = signal_out(3:end);\n\nfigure(85)\ntitle('Amplification')\nplot(after_gain_control./before_gain_control)\n\nfigure(75)\nplot(real(before_gain_control))\n\nfigure(83)\nplot(real(after_gain_control))\n\n\n%signal_out = \n\n%signal_out = zeros(1,N);\n%for i = 1:N\n      %      distance = abs(symbols(i) - theta);\n   %[emp,index_2] =min(distance);\n    \n%    signal_out = [signal_out bitmap(index_2,1) bitmap(index_2,2) bitmap(index_2,3) bitmap(index_2,4)];\n   %  signal_out = [signal_out bitmap(index_2,:)];\n%end\n\n\n%test(:,1) = signal_out;\n%test(:,2) = bits;\ntest_2 = bits;\n%test(:,2) = bits;\n\nN = length(symbols);\nstart_index = start_index;\nr1 = bits;\nr2 = signal_out;\nr3 = symbols;\n\n\n%error = sum(abs(bits(index_test:index_test) - signal_out));\nfigure(26)\nplot(symbols,'.')\ntitle('synchronized symbol constellation')\n%stop = min(10000,length(signal_out));\n\n\n%stop = min(length(signal_out),length(bits))-10000;\nstop = 50000;\nerror = sum(abs(bits(1:stop) - signal_out(1:stop))); % Test Fredrik\nfigure(27)\nplot(real(symbols(1:stop/4)),'r')\nhold on\nplot(real(bit_sym))\nlength_signal_out = length(signal_out);\nbit_error_rate = error./stop;\n\n\nfigure(95)\nplot(symbols(2000:end))\ntitle('test result')\n\nfigure(951)\nplot(symbols(10000:50000),'.')"("start_index"=w94, "bits"=w64, "symbols"=w93, "bit_sym"=w63, "before_gain_control"=w49, "after_gain_control"=w48) -> ("bit_error_rate"=→"bit_error_rate":dbl, "length_signal_out"=→"length_signal_out":i32, "signal_out"=w74:i32[], "error"=→"error":dbl)  [unwired: 1 in, 2 out]
  n70 = Array Size(array=w64) -> (size(s)=→"size(s)":i32)
  n71 = Not Equal To 0?(x=w74) -> (x != 0?=w72:bool[])
  n72 = call "write_to_file.vi"("data 3"=w72, "file (use dialog) in"="file (use dialog) 2") -> ()  [unwired: 10 in]
